vi "meter-1.vi"() -> ()   [LabVIEW 2010]
uses:
  VarableID.ctl
panel:
  out "Data 2":string
  out "Data1":string
  in  "视在功率":bool
  in  "功率因数":bool
  in  "电压":bool
  in  "电流":bool
  in  "Port2":refnum<visa-resource-name>="COM1" caption="端口号"
  in  "baud rate":u32=2400 caption="波特率"
  in  "退出系统":bool
  in  "软件使用说明":bool
  out "?":dbl[](graph)
  in  "IP地址设置":string="010000000000"
  out "初始化状态":bool
  in  "启动采集":bool=TRUE
  in  "初始化":bool
  in  "Port1":refnum<visa-resource-name>="COM1" caption="端口号"
  # "智能电表信息采集系统"
  # "端口参数设置"
  # "信号采集选项"
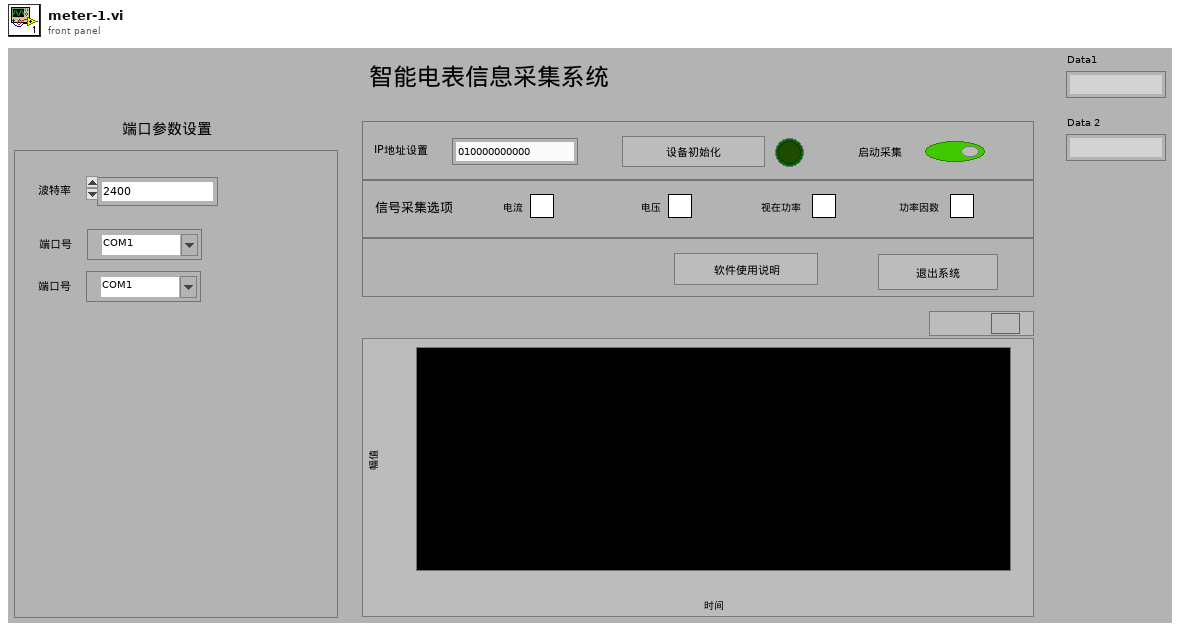
[diagram p1: front panel]
types:
  T1 = typedef "VarableID.ctl" = enum16{"current", "voltage", "power", "PF"}
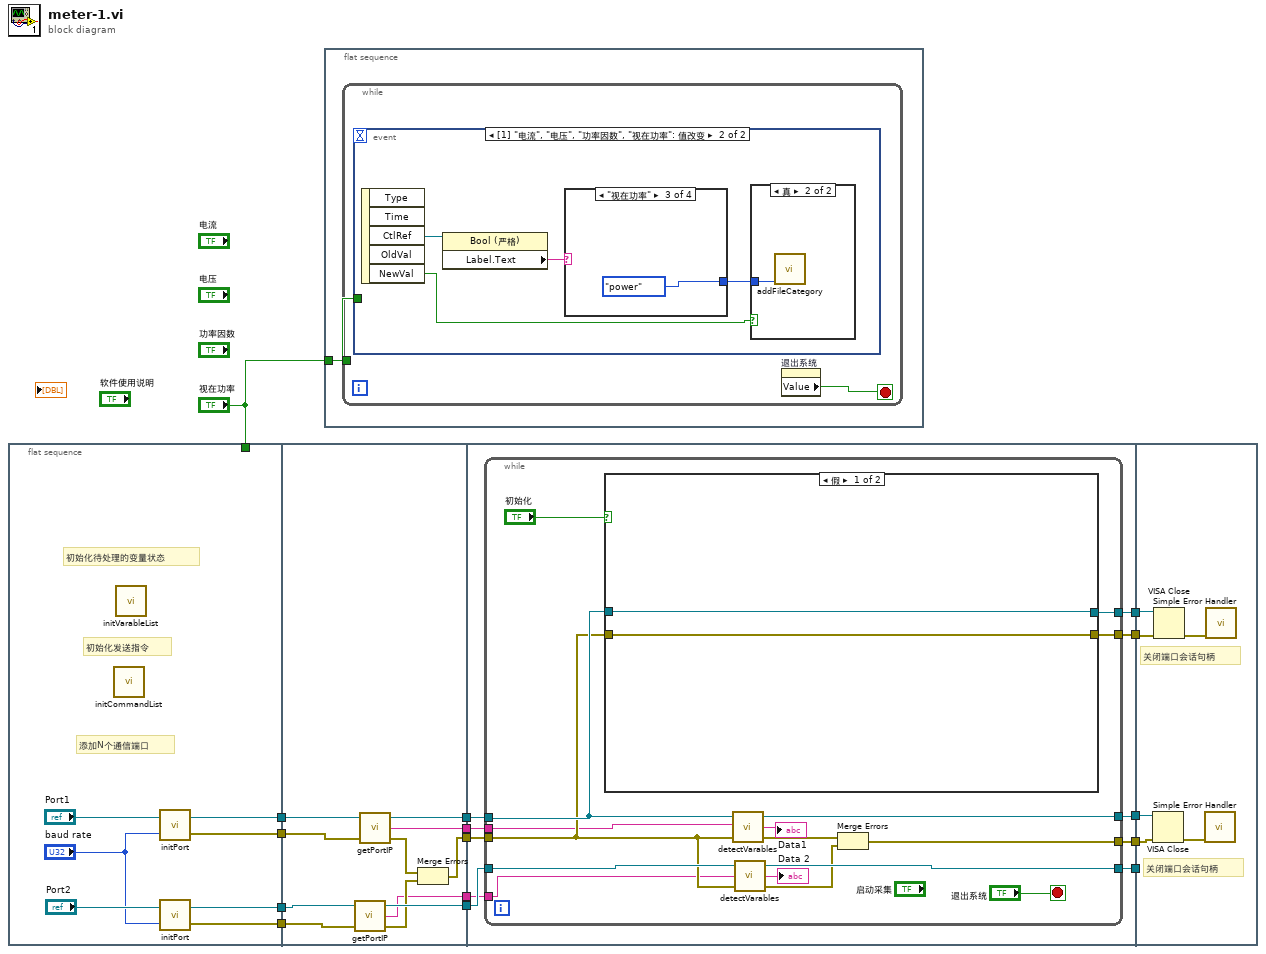
[diagram p0: block diagram]
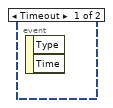
[diagram p2: hidden frame]
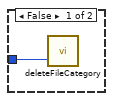
[diagram p3: hidden frame]
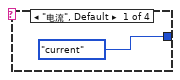
[diagram p4: hidden frame]
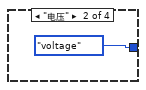
[diagram p5: hidden frame]
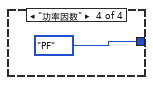
[diagram p6: hidden frame]
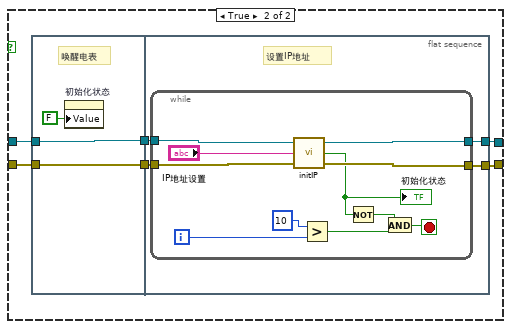
[diagram p7: hidden frame]
diagram:
  n1 = flat-sequence {
    tunnel: [w21] -> w8
    tunnel: [w18] -> w6
    tunnel: "视在功率" -> [_]
    tunnel: [w17] -> w4
    tunnel: [w16] -> w3
    tunnel: [w25] -> w9
    tunnel: w8 -> [w27]
    tunnel: [w26] -> w7
    tunnel: w6 -> [w30]
    tunnel: [w29] -> w5
    tunnel: w4 -> [w33]
    tunnel: w3 -> [w31]
    tunnel: [w24] -> w2
    tunnel: [w23] -> w1
    tunnel: w9 -> [w42]
    tunnel: w7 -> [w43]
    tunnel: [w41] -> w15
    tunnel: [w40] -> w14
    tunnel: [w39] -> w13
    tunnel: [w38] -> w12
    tunnel: w5 -> [w37]
    tunnel: [w36] -> w11
    tunnel: w2 -> [w35]
    tunnel: w1 -> [w34]
    tunnel: w15 -> [w89]
    tunnel: w14 -> [w88]
    tunnel: w13 -> [w87]
    tunnel: w12 -> [w86]
    tunnel: w11 -> [_]
    frame #0 {
      # "初始化发送指令"
      # "添加N个通信端口"
      # "初始化待处理的变量状态"
      n2 = call "initCommandList.vi"() -> ()  [unwired: 12 in]
      n3 = call "initVarableList.vi"() -> ()  [unwired: 12 in]
      n4 = call "initPort.vi"("baud rate"="baud rate", "VISA resource name"="Port1") -> ("error out"=w17:errorcluster, "reference out"=w21:refnum<visa-resource-name>)
      n5 = call "initPort.vi"("baud rate"="baud rate", "VISA resource name"="Port2") -> ("error out"=w16:errorcluster, "reference out"=w18:refnum<visa-resource-name>)
    }
    frame #1 {
      n6 = call "getPortIP.vi"("error in (no error)"=w31, "VISA resource name"=w30) -> ("error out"=w28:errorcluster, "portIP"=w23:string, "VISA resource name 2"=w29:refnum<visa-resource-name>)  [unwired: 1 in]
      n7 = call "getPortIP.vi"("error in (no error)"=w33, "VISA resource name"=w27) -> ("error out"=w32:errorcluster, "portIP"=w24:string, "VISA resource name 2"=w26:refnum<visa-resource-name>)  [unwired: 1 in]
      n8 = Merge Errors(w32, w28) -> (w25:errorcluster)
    }
    frame #2 {
      n9 = while {
        tunnel: [w59] -> w41
        tunnel: [w58] -> w40
        tunnel: w43 -> [w55]
        tunnel: w42 -> [w52]
        tunnel: [w54] -> w39
        tunnel: [w48] -> w38
        tunnel: w37 -> [w53]
        tunnel: [w51] -> w36
        tunnel: w35 -> [w47]
        tunnel: w34 -> [w46]
        stop <- "退出系统" stop-if-true
        n10 = case shown="假" "初始化" {
          tunnel: w55 -> [w61 w67]
          tunnel: w52 -> [w60 w66]
          tunnel: [w61 w63] -> w59
          tunnel: [w60 w62] -> w58
          frame False {
          }
          frame True {
            n11 = flat-sequence {
              tunnel: w67 -> [w69]
              tunnel: w66 -> [w68]
              tunnel: [w69] -> w65
              tunnel: [w68] -> w64
              tunnel: w65 -> [w74]
              tunnel: w64 -> [w73]
              tunnel: [w72] -> w63
              tunnel: [w71] -> w62
              frame #0 {
                # "唤醒电表"
                n12 = property on="初始化状态" class="Bool (严格)"("Value"=FALSE ("初始化状态")) -> ()  [unwired: 2 in, 2 out]
              }
              frame #1 {
                # "设置IP地址"
                n13 = while {
                  tunnel: w74 -> [w81]
                  tunnel: w73 -> [w80]
                  tunnel: [w79] -> w72
                  tunnel: [w78] -> w71
                  i -> [w83]
                  stop <- w82 stop-if-true
                  n14 = call "initIP.vi"("error in"=w80, "IP Address"="IP地址设置", "reference in"=w81) -> ("error out"=w78:errorcluster, "初始化状态"=w75:bool, "reference out"=w79:refnum<visa-resource-name>)
                  "初始化状态" <- w75
                  n15 = Greater?(x=10, y=w83) -> (0:w85:bool)
                  n16 = Not(x=w75) -> (.not. x?=w76:bool)
                  n17 = And(x=w76, y=w85) -> (x .and. y?=w82:bool)
                }
              }
            }
          }
        }
        n18 = call "detectVarables.vi"("error in (no error)"=w52, "PortIP"=w47, "VISA resource name"=w55) -> ("error out"=w50:errorcluster, "Data"=→"Data1":string, "VISA resource name 2"=w54:refnum<visa-resource-name>)
        n19 = call "detectVarables.vi"("error in (no error)"=w52, "PortIP"=w46, "VISA resource name"=w53) -> ("error out"=w49:errorcluster, "Data"=→"Data 2":string, "VISA resource name 2"=w51:refnum<visa-resource-name>)
        n20 = Merge Errors(w50, w49) -> (w48:errorcluster)
      }
    }
    frame #3 {
      # "关闭端口会话句柄"
      # "关闭端口会话句柄"
      n21 = VISA Close(VISA resource name=w87, error in (no error)=w86) -> (error out=w90:errorcluster)
      n22 = VISA Close(VISA resource name=w89, error in (no error)=w88) -> (error out=w91:errorcluster)
      n23 = call <vilib>:"Simple Error Handler.vi"("error in (no error)"=w90) -> ()  [unwired: 1 in, 8 out]
      n24 = call <vilib>:"Simple Error Handler.vi"("error in (no error)"=w91) -> ()  [unwired: 1 in, 8 out]
    }
  }
  n25 = flat-sequence {
    tunnel: "视在功率" -> [w92]
    frame #0 {
      n26 = while {
        tunnel: w92 -> [w94]
        stop <- w93 stop-if-true
        n27 = event shown="[1] \"电流\", \"电压\", \"功率因数\", \"视在功率\": 值改变" {
          selector: _ -> [_ _]
          dyn-events: _ -> [_ _]
          timeout: _ -> [_ _]
          tunnel: w94 -> [_ _]
          event Timeout {
            n28 = event-data() -> ()  [unwired: 1 in, 2 out]
          }
          event "电流", "电压", "功率因数", "视在功率": Value Change {
            n29 = event-data() -> ("CtlRef"=w95:refnum<vi>, "NewVal"=w96:bool)  [unwired: 1 in, 3 out]
            n30 = property class="Bool (严格)"(reference=w95) -> ("Label.Text"=w98:string)  [unwired: 1 in, 2 out]
            n31 = case shown="\"视在功率\"" w98 {
              tunnel: [VarableID."current" ("VarableID") VarableID."voltage" ("VarableID") VarableID."power" ("VarableID") VarableID."PF" ("VarableID")] -> w97
              frame "电流", Default {
              }
              frame "电压" {
              }
              frame "视在功率" {
              }
              frame "功率因数" {
              }
            }
            n32 = case shown="真" w96 {
              tunnel: w97 -> [w99 w100]
              frame False {
                n33 = call "deleteFileCategory.vi"("VarableID"=w99) -> ()  [unwired: 2 in]
              }
              frame True {
                n34 = call "addFileCategory.vi"("VarableID"=w100) -> ()  [unwired: 2 in]
              }
            }
          }
        }
        n35 = property on="退出系统" class="Bool (严格)"() -> ("Value"=w93:bool)  [unwired: 2 in, 2 out]
      }
    }
  }
